vi "observe.vi"(8 "error in (no error)":errorcluster, 11 "controller in":refnum<class "controller.lvclass">) -> (0 "error out":errorcluster, 2 "State":dbl, 3 "controller out":refnum<class "controller.lvclass">)   [LabVIEW 2025, in "controller.lvclass"]
uses:
  controller.lvclass
  controller.lvclass/controller.ctl
  <vilib>/DAQmx/read.llb/DAQmx Read (Analog DBL 1Chan 1Samp).vi
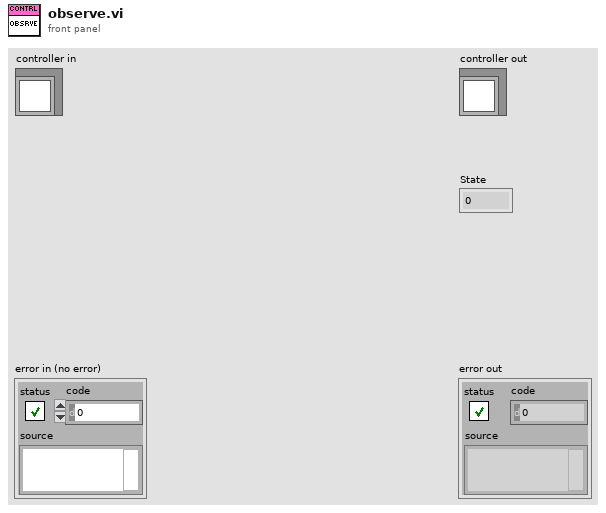
[diagram p1: front panel]
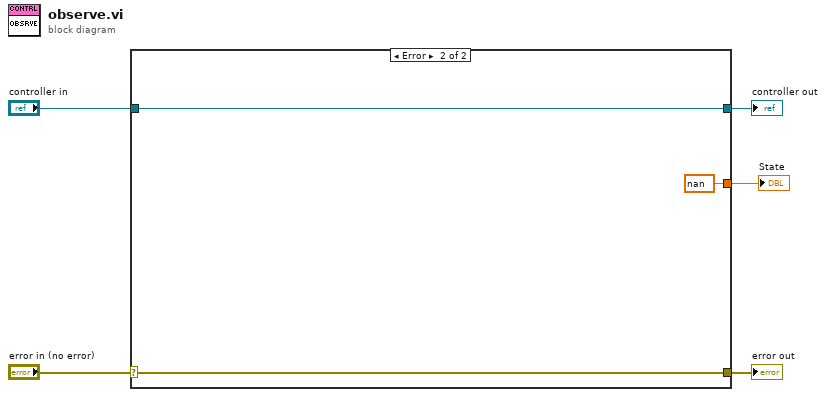
[diagram p0: block diagram]
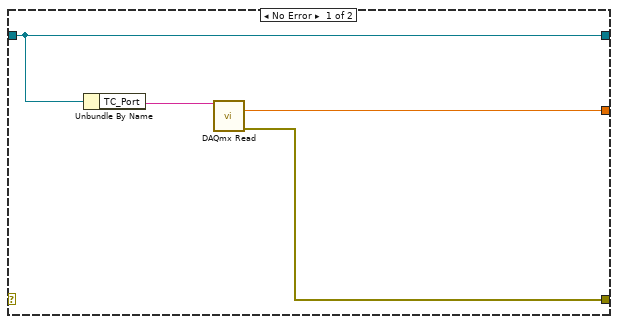
[diagram p2: hidden frame]
diagram:
  n1 = case shown="Error" "error in (no error)" {
    selector: "error in (no error)" -> [_ w12]
    tunnel: [w6 w12] -> w4
    tunnel: [w9 w11] -> w2
    tunnel: "controller in" -> [w9 w11]
    tunnel: [w7 nan ("data")] -> w1
    frame No Error {
      n2 = Unbundle By Name(w9) -> ("TC_Port"=w8:string)
      n3 = call-poly <vilib>:"DAQmx Read.vi"("task/channels in"=w8) -> ("data"=w7:dbl, "error out"=w6:errorcluster)  [unwired: 12 in, 1 out]
    }
    frame Error {
    }
  }
  "error out" <- w4
  "controller out" <- w2
  "State" <- w1
